vi "CameraLoader.vi"() -> ()   [LabVIEW 2024]
uses:
  <vilib>/userDefined/High Color/IMAQdx.ctl
  <vilib>/vision/driver/NI_Vision_Acquisition_Software.lvlib
panel:
  in  "Cam No.":T1
  in  "stop":bool
  out "Image Out":T2(plugin-control)
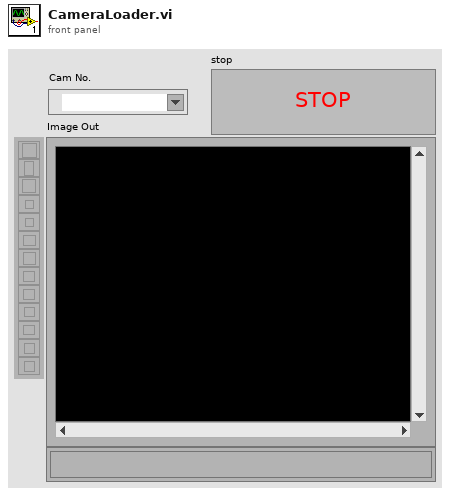
[diagram p1: front panel]
types:
  T1 = typedef "IMAQdx.ctl" = refnum<k21>
  T2 = typedef "IMAQ Image.ctl" = refnum<image>
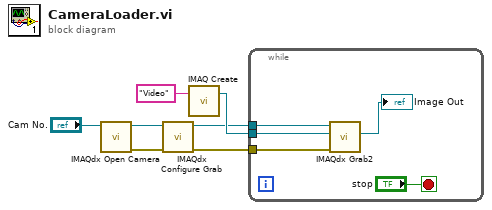
[diagram p0: block diagram]
diagram:
  n1 = call <vilib>:"IMAQdx Open Camera.vi"("Session In"="Cam No.") -> ("error out"=w3:errorcluster, "Session Out"=w4:T1)  [unwired: 9 in]
  n2 = call <vilib>:"IMAQdx Configure Grab.vi"("error in"=w3, "Session In"=w4) -> ("error out"=w1:errorcluster, "Session Out"=w2:T1)  [unwired: 8 in]
  n3 = call "IMAQ Create"("Image Name"="Video") -> ("New Image"=w6:T2)  [unwired: 4 in, 1 out]
  n4 = while {
    tunnel: w1 -> [w9]
    tunnel: w6 -> [w11]
    tunnel: w2 -> [w8]
    stop <- "stop" stop-if-true
    n5 = call <vilib>:"IMAQdx Grab2.vi"("error in"=w9, "Image In"=w11, "Session In"=w8) -> ("Image Out"=→"Image Out":T2)  [unwired: 5 in, 3 out]
  }
